vi "Do.vi"(8 "error in (no error)":errorcluster, 10 "Actor in":refnum<class "Actor.lvclass">, 11 "Write Card# Msg":refnum<class "Write Card# Msg.lvclass">) -> (0 "error out":errorcluster, 2 "Actor out":refnum<class "Actor.lvclass">)   [LabVIEW 2012, in "Display Panel.lvlib" / "Write Card# Msg.lvclass"]
doc: "This VI delivers the message to the actor by calling the appropriate method(s) on the actor."
uses:
  Write Card# Msg.lvclass
  <vilib>/ActorFramework/Actor/Actor.lvclass
  Power Meter Display/Power Meter Display.lvclass
  Write Card# Msg.lvclass/Write Card# Msg.ctl
  Abstract Display/Abstract Display.lvclass
panel:
  out "Card#":dbl
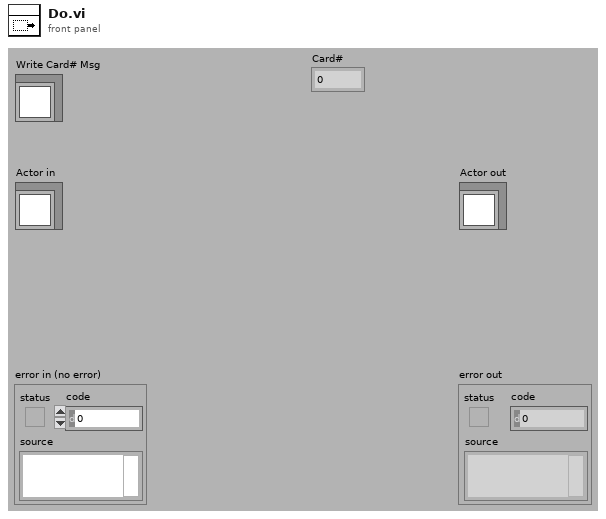
[diagram p1: front panel]
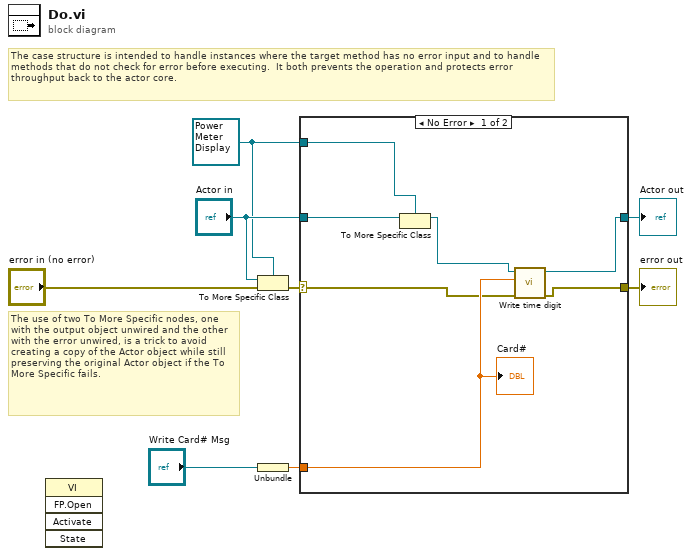
[diagram p0: block diagram]
diagram:
  w2 = refnum<class "Power Meter Display.lvclass"> refnum ("Actor in")
  # "The use of two To More Specific nodes, one with the output object unwired and the other with the error unwired, is a trick to avoid creating a copy of the Actor object while still preserving the original Actor object if the To More Specific fails."
  # "The case structure is intended to handle instances where the target method has no error input and to handle methods that do not check for error before executing.  It both prevents the operation and protects error throughput back to the actor core."
  n1 = invoke class="VI" method="FP.Open"() -> ()  [unwired: 5 in, 5 out]
  n2 = To More Specific Class(target class=w2, reference="Actor in", error in="error in (no error)") -> (error out=w6:errorcluster)  [unwired: 1 out]
  n3 = Unbundle("Write Card# Msg") -> (w1:dbl)
  n4 = case shown="No Error" w6 {
    selector: w6 -> [w10 w17]
    tunnel: [w9 w17] -> w5
    tunnel: [w12 w16] -> w4
    tunnel: "Actor in" -> [w15 w16]
    tunnel: w2 -> [w14 _]
    tunnel: w1 -> [w11 _]
    frame No Error {
      n5 = To More Specific Class(target class=w14, reference=w15) -> (specific class reference=w13:refnum<class "Power Meter Display.lvclass">)  [unwired: 1 in, 1 out]
      n6 = call "Write time digit.vi"("error in (no error)"=w10, "Time"=w11, "Abstract Display in"=w13) -> ("error out"=w9:errorcluster, "Abstract Display out"=w12:refnum<class "Power Meter Display.lvclass">)  [unwired: 7 in]
      "Card#" <- w11
    }
    frame Error {
      # "If type check fails, pass the original object out again."
    }
  }
  "error out" <- w5
  "Actor out" <- w4
